vi "Test Boolean Logic.vi"() -> ()   [LabVIEW 2021]
uses:
  Source/Functions/Logic/Support/NOT/Bool/Method.vi
  Source/Functions/Logic/Support/EXNOR/Bool/Method.vi
  Source/Functions/Logic/Support/NOR/Bool/Method.vi
  Source/Functions/Logic/Support/OR/Bool/Method.vi
  Source/Functions/Logic/Support/AND/Bool/Method.vi
  Source/Functions/Logic/Support/EXOR/Bool/Method.vi
  Source/Abs_Types/Boolean/Abs_Boolean.lvclass
  Source/Constants/Support/Bool/Const_Bool.lvclass
  Source/Functions/Logic/Support/NOT/Bool/NOT_Bool.lvclass
  Source/Functions/Logic/Support/EXOR/Bool/EXOR_Bool.lvclass
  Source/Functions/Logic/Support/AND/Bool/AND_Bool.lvclass
  Source/Functions/Logic/Support/OR/Bool/OR_Bool.lvclass
  Source/Functions/Logic/Support/NOR/Bool/NOR_Bool.lvclass
  Source/Functions/Logic/Support/EXNOR/Bool/EXNOR_Bool.lvclass
panel:
  out "EXNOR":bool
  out "NOR":bool
  out "OR":bool
  out "AND":bool
  out "EXOR":bool
  in  "Boolean 3":bool
  in  "Boolean 2":bool
  out "Not":bool
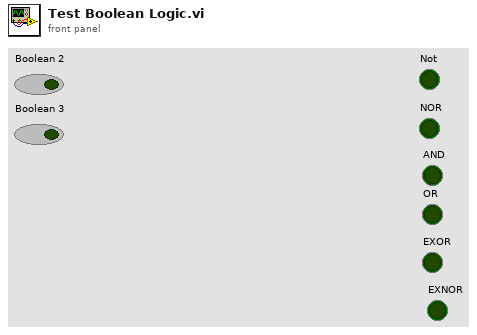
[diagram p1: front panel]
types:
  T1 = typedef "EXNOR_Bool.lvclass/Abs_Type.ctl" = refnum<class "Abs_Boolean.lvclass">
  T2 = typedef "EXOR_Bool.lvclass/Abs_Type.ctl" = refnum<class "Abs_Boolean.lvclass">
  T3 = typedef "NOR_Bool.lvclass/Abs_Type.ctl" = refnum<class "Abs_Boolean.lvclass">
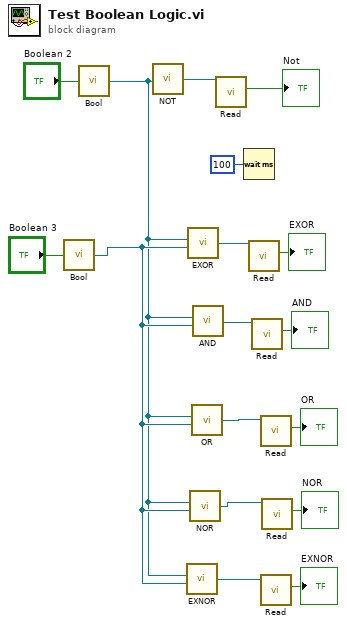
[diagram p0: block diagram]
diagram:
  n1 = call "Bool.vi"("Boolean"="Boolean 3") -> ("Abs_Boolean.lvclass"=w4:refnum<class "Abs_Boolean.lvclass">)  [unwired: 4 in]
  n2 = call "Bool.vi"("Boolean"="Boolean 2") -> ("Abs_Boolean.lvclass"=w1:refnum<class "Abs_Boolean.lvclass">)  [unwired: 4 in]
  n3 = call-poly "NOT.vi"("Bool"=w1) -> ("Result"=w17:refnum<class "Abs_Boolean.lvclass">)  [unwired: 4 in]
  n4 = call-poly "EXNOR.vi"("B"=w4, "A"=w1) -> ("Result"=w2:T1)  [unwired: 4 in]
  n5 = call-poly "EXOR.vi"("B"=w4, "A"=w1) -> ("Result"=w12:T2)  [unwired: 4 in]
  n6 = call-poly "NOR.vi"("B"=w4, "A"=w1) -> ("Result"=w5:T3)  [unwired: 4 in]
  n7 = call-poly "OR.vi"("B"=w4, "A"=w1) -> ("Result"=w7:refnum<class "Abs_Boolean.lvclass">)  [unwired: 4 in]
  n8 = call-poly "AND.vi"("B"=w4, "A"=w1) -> ("Result"=w9:refnum<class "Abs_Boolean.lvclass">)  [unwired: 4 in]
  n9 = call-dynamic "Read.vi"("Boolean in"=w17) -> ("Boolean"=→"Not":bool)  [unwired: 8 in, 2 out]
  n10 = Wait (ms)(milliseconds to wait=u32 100) -> ()  [unwired: 1 out]
  n11 = call-dynamic "Read.vi"("Boolean in"=w12) -> ("Boolean"=→"EXOR":bool)  [unwired: 8 in, 2 out]
  n12 = call-dynamic "Read.vi"("Boolean in"=w9) -> ("Boolean"=→"AND":bool)  [unwired: 8 in, 2 out]
  n13 = call-dynamic "Read.vi"("Boolean in"=w7) -> ("Boolean"=→"OR":bool)  [unwired: 8 in, 2 out]
  n14 = call-dynamic "Read.vi"("Boolean in"=w2) -> ("Boolean"=→"EXNOR":bool)  [unwired: 8 in, 2 out]
  n15 = call-dynamic "Read.vi"("Boolean in"=w5) -> ("Boolean"=→"NOR":bool)  [unwired: 8 in, 2 out]
